vi "Get Macro Configs.vi"(8 "error in (no error)":errorcluster, 11 "Motions Configuration in":refnum<class "Motions Configuration.lvclass">) -> (0 "error out":errorcluster, 2 "Array of Macro Configs":T1[](array[typedef]), 3 "Motions Configuration out":refnum<class "Motions Configuration.lvclass">)   [LabVIEW 2016, in "Hardware.lvlib" / "Motions.lvlib" / "Motions Configuration.lvclass"]
uses:
  <userlib>/Common Components/Hardware/Abstract System/Motions/Motions Config/Motions Configuration.lvclass
  <userlib>/Common Components/Hardware/Abstract System/Motions/Motions Config/Macro Config.ctl
  <userlib>/Common Components/TriggerAction Q/TriggerAction Q/Element Data.ctl
  <userlib>/Common Components/Hardware/Abstract System/Motions/Motions Config/Motions Configuration.lvclass/Motions Configuration.ctl
  <userlib>/Common Components/Hardware/Abstract System/Motions/Motions/Motions.lvclass/Motions.ctl
  <userlib>/Common Components/TriggerAction Q/TriggerAction Q/TriggerAction Q.lvclass
  <userlib>/Common Components/Hardware/Abstract System/Motions/Motions/Motions.lvclass
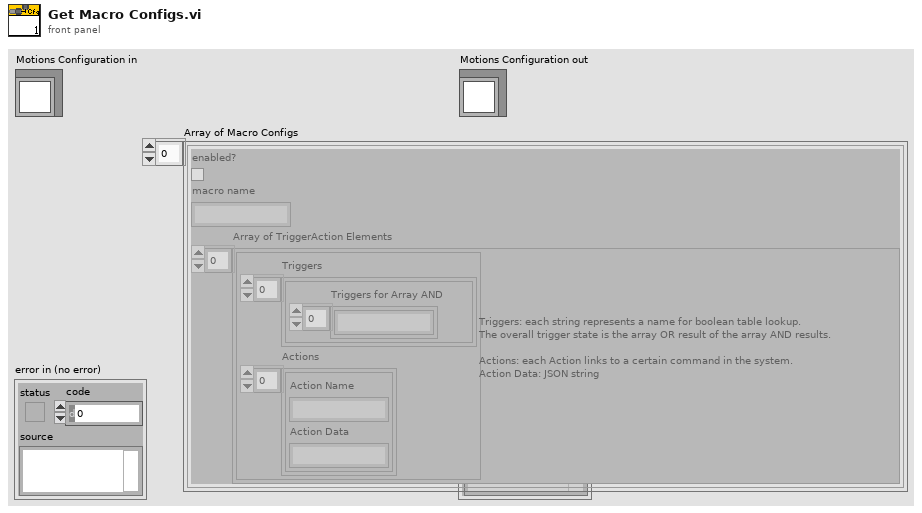
[diagram p1: front panel]
types:
  T1 = typedef "Hardware.lvlib/Motions.lvlib/Motions Configuration.lvclass/Macro Config.ctl" = cluster{"enabled?":bool, "macro name":string, "Array of TriggerAction Elements":T2[]}
  T2 = typedef "TriggerAction Q.lvclass/Element Data.ctl" = cluster{"Triggers":cluster{"Triggers for Array AND":string[]}[], "Actions":cluster{"Action Name":string, "Action Data":string}[]}
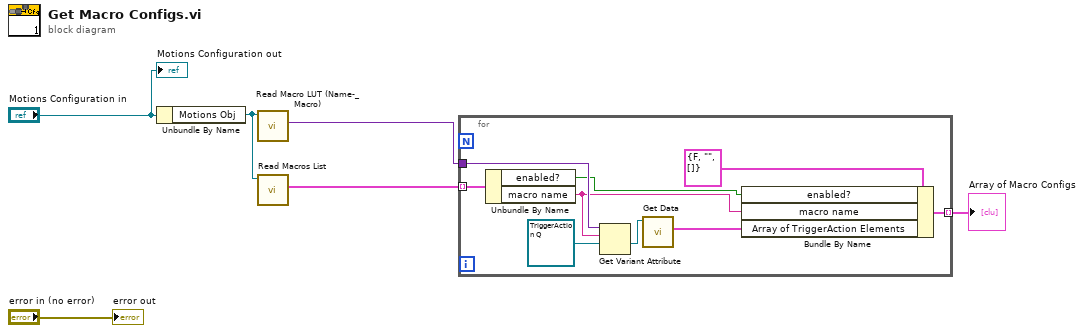
[diagram p0: block diagram]
diagram:
  n1 = Unbundle By Name("Motions Configuration in") -> ("Motions Obj"=w4:refnum<class "Motions.lvclass">)
  n2 = call <userlib>:"Read Macro LUT (Name-_Macro).vi"("Motions in"=w4) -> ("Macro LUT (Name->Macro)"=w2:variant)  [unwired: 9 in, 1 out]
  n3 = call <userlib>:"Read Macros List.vi"("Motions in"=w4) -> ("Macros List"=w3:cluster{"enabled?":bool, "macro name":string}[])  [unwired: 9 in, 1 out]
  n4 = for {
    tunnel: w3 -> [w15] mode=indexing
    tunnel: w2 -> [w14]
    tunnel: [w7] -> w1 mode=indexing
    n5 = Unbundle By Name(w15) -> ("enabled?"=w10:bool, "macro name"=w9:string)
    n6 = Get Variant Attribute(Variant=w14, name=w9, default value (empty Variant)=refnum<class "TriggerAction Q.lvclass"> refnum ("TriggerAction Q.lvclass")) -> (value=w12:refnum<class "TriggerAction Q.lvclass">)  [unwired: 1 in, 3 out]
    n7 = call <userlib>:"Get Data.vi"("TriggerAction in"=w12) -> ("Array of TriggerAction Elements"=w8:T2[])  [unwired: 8 in, 2 out]
    n8 = Bundle By Name(cluster=T1 {"enabled?"=FALSE, "macro name"="", "Array of TriggerAction Elements"=[]} ("Cluster"), "enabled?"=w10, "macro name"=w9, "Array of TriggerAction Elements"=w8) -> (w7:T1)
  }
  "Array of Macro Configs" <- w1
  "error out" <- "error in (no error)"
  "Motions Configuration out" <- "Motions Configuration in"
